vi "Recursive Find LVClasses.vi"(8 "error in (no error)":errorcluster, 11 "reference":refnum<vi>) -> (0 "error out":errorcluster, 3 "Class References":refnum<vi>[](array[refnum]))   [LabVIEW 2020, in "Process Generation.lvlib" / "New Class Dialog.lvclass"]
uses:
  New Class Dialog.lvclass
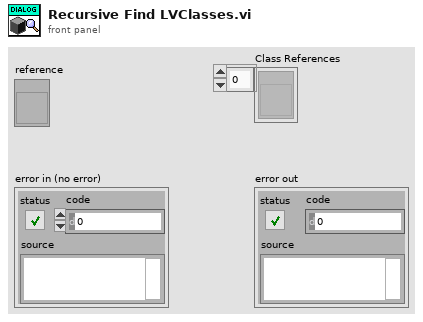
[diagram p1: front panel]
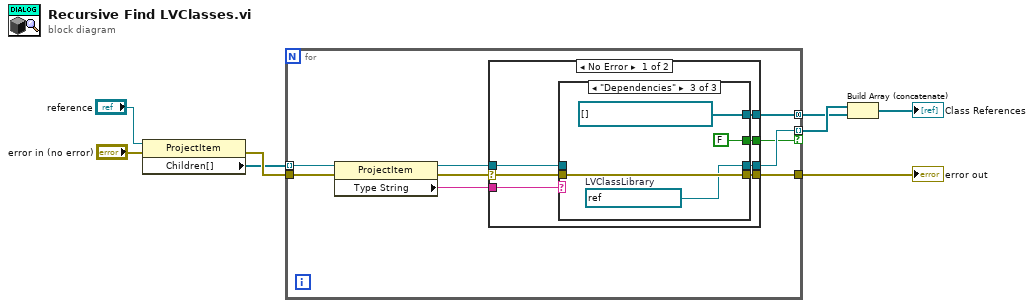
[diagram p0: block diagram]
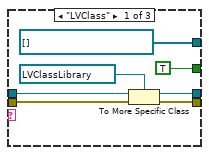
[diagram p2: hidden frame]
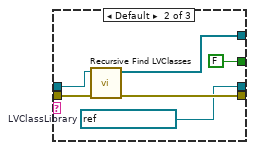
[diagram p3: hidden frame]
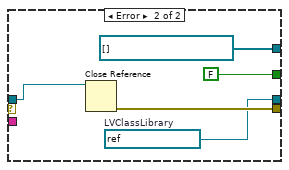
[diagram p4: hidden frame]
diagram:
  n1 = property class="ProjectItem"(reference="reference", error in="error in (no error)") -> (error out=w6:errorcluster, "Children[]"=w4:refnum<vi>[])  [unwired: 1 out]
  n2 = for {
    tunnel: w4 -> [w17] mode=indexing
    tunnel: [w12] -> w7 mode=indexing if=w11
    tunnel: w6 -> [w16]
    tunnel: [w14] -> w8
    tunnel: [w10] -> w1 mode=concatenating
    n3 = property class="ProjectItem"(reference=w17, error in=w16) -> (reference out=w13:refnum<vi>, error out=w15:errorcluster, "Type String"=w9:string)
    n4 = case shown="No Error" w15 {
      selector: w15 -> [w24 _]
      tunnel: [w23 w45] -> w14
      tunnel: w13 -> [w22 w46]
      tunnel: [w21 w42] -> w12
      tunnel: w9 -> [w20 _]
      tunnel: [w19 FALSE] -> w11
      tunnel: [w18 refnum<vi>[] [] ("Class References")] -> w10
      frame No Error {
        n5 = case shown="\"Dependencies\"" w20 {
          tunnel: w24 -> [w26 w37 w41]
          tunnel: [w27 w36 w41] -> w23
          tunnel: w22 -> [w31 w35 _]
          tunnel: [w28 w32 w39] -> w21
          tunnel: [TRUE FALSE FALSE] -> w19
          tunnel: [refnum<vi>[] [] ("Class References") w34 refnum<vi>[] [] ("Class References")] -> w18
          frame "LVClass" {
            n6 = To More Specific Class(target class=refnum<vi> refnum ("Class References"), reference=w31, error in=w26) -> (specific class reference=w28:refnum<vi>, error out=w27:errorcluster)
          }
          frame Default {
            w32 = refnum<vi> refnum  # LVClassLibrary
            n7 = call "Recursive Find LVClasses.vi"("error in (no error)"=w37, "reference"=w35) -> ("error out"=w36:errorcluster, "Class References"=w34:refnum<vi>[])  [unwired: 8 in]
          }
          frame "Dependencies" {
            w39 = refnum<vi> refnum  # LVClassLibrary
          }
        }
      }
      frame Error {
        w42 = refnum<vi> refnum  # LVClassLibrary
        n8 = Close Reference(reference=w46) -> (error out=w45:errorcluster)  [unwired: 1 in]
      }
    }
  }
  "error out" <- w8
  n9 = Build Array (concatenate)(w7, w1) -> (→"Class References":refnum<vi>[])
